vi "Periodic Tasks.vi"(8 "error in":errorcluster) -> ()   [LabVIEW 2017]
doc: "This VI runs in parallel to other tasks. It can contain as many user-defined periodic loops as you need. These can carry out PID or other sorts of timed response."
uses:
  <vilib>/Rock Robotics/WPI/Utilities/WPI_GetSetVariantRefNum.vi
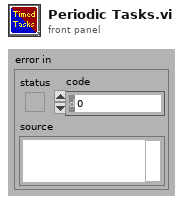
[diagram p1: front panel]
types:
  T1 = typedef "WPI_JoystickDevRef.ctl" = cluster{"Device":T2}
  T2 = typedef "WPI_JoystickDeviceEnum.ctl" = enum16{"USB 0", "USB 1", "USB 2", "USB 3", "USB 4", "USB 5"}
  T3 = typedef "WPI_RobotDriveDevRef.ctl" = cluster{"DevStatus":errorcluster, "Motors[]":T4[], "Square Inputs":bool, "Max Output":dbl}
  T4 = typedef "WPI_MotorControlDeviceRef.ctl" = cluster{"DeviceStatus":errorcluster, "Type":T5, "PWM":cluster{"PWM Channel":T6, "DeadBand":T7}, "CAN":cluster{"Device Number":u8, "SetOutput VI Ref":variant, "GetOutput VI Ref":variant, "Enable VI Ref":variant, "Disable VI Ref":variant, "Data":variant}, "Invert":bool, "DIO PWM":cluster{"PWM \"Enable\" Channel":T6, "DIOChannel":T8, "PWM Rate":dbl}}
  T5 = typedef "WPI_MotorControlType.ctl" = enum16{"PWM", "CAN", "DIO PWM"}
  T6 = typedef "FPGA_DIOPWMChannel.ctl" = enum8{"PWM 0", "PWM 1", "PWM 2", "PWM 3", "PWM 4", "PWM 5", "PWM 6", "PWM 7", "PWM 8", "PWM 9", "PWM MXP 0", "PWM MXP 1", "PWM MXP 2", "PWM MXP 3", "PWM MXP 4", "PWM MXP 5", "PWM MXP 6", "PWM MXP 7", "PWM MXP 8", "PWM MXP 9", "Invalid"}
  T7 = typedef "WPI_PWMDeadband.ctl" = cluster{"Name":string, "maxPositivePwm":i32, "minPositivePwm":i32, "centerPwm":i32, "maxNegativePwm":i32, "minNegativePwm":i32, "angularRange":u16}
  T8 = typedef "FPGA_DIOChannel.ctl" = enum8{"DIO 0", "DIO 1", "DIO 2", "DIO 3", "DIO 4", "DIO 5", "DIO 6", "DIO 7", "DIO 8", "DIO 9", "DIO MXP 0", "DIO MXP 1", "DIO MXP 2", "DIO MXP 3", "DIO MXP 4", "DIO MXP 5", "DIO MXP 6", "DIO MXP 7", "DIO MXP 8", "DIO MXP 9", "DIO MXP 10", "DIO MXP 11", "DIO MXP 12", "DIO MXP 13", "DIO MXP 14", "DIO MXP 15", "SPI Port CS1", "SPI Port CS2", "SPI Port CS3", "SPI Port MISO", "SPI Port MOSI", "Invalid"}
  T9 = cluster{"JoystickDevRef":T1, "RobotDriveDevRef":T3}
  T10 = typedef "WPI_I2CDevRef.ctl" = cluster{"DevStatus":errorcluster, "Device Address":u8, "Handle":i32, "I2C Bus":T11}
  T11 = typedef "i2c_bus.ctl" = enum16{"I2C On-Board", "I2C MXP", "Invalid"}
  T12 = typedef "WPI_DriverStationRobotMode2.ctl" = enum16{"Autonomous Disabled", "Autonomous Enabled", "Teleop Disabled", "Teleop Enabled", "Disconnected", "Finish", "Test Disabled", "Test Enabled", "Emergency Stopped"}
  T13 = typedef "WPI_DriverStationAllianceInfo.ctl" = enum16{"Red", "Blue", "Invalid"}
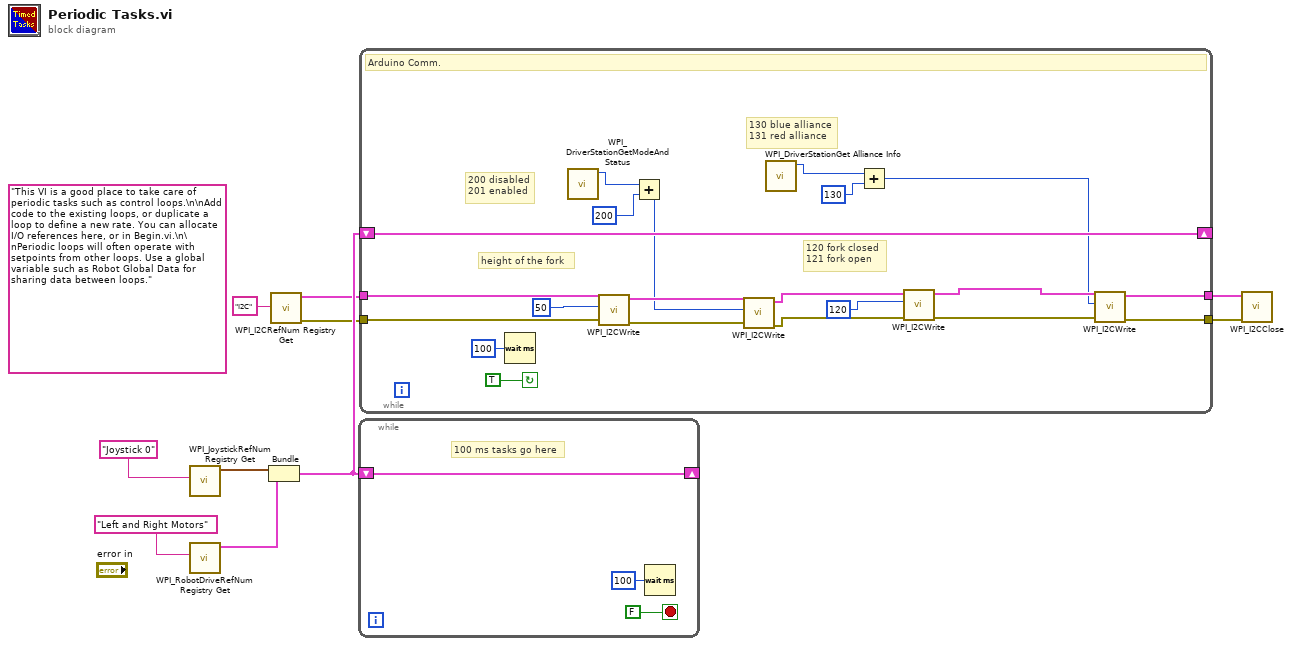
[diagram p0: block diagram]
diagram:
  (unwired) "This VI is a good place to take care of periodic tasks such as control loops.\n\nAdd code to the existing loops, or duplicate a loop to define a new rate. You can allocate I/O references here, or in Begin.vi.\n\nPeriodic loops will often operate with setpoints from other loops. Use a global variable such as Robot Global Data for sharing data between loops."
  n1 = call <vilib>:"WPI_JoystickRefNum Registry Get.vi"("refnum name"="Joystick 0") -> ("JoystickDevRef"=w8:T1)  [unwired: 1 in, 9 out]
  n2 = call <vilib>:"WPI_RobotDriveRefNum Registry Get.vi"("refnum name"="Left and Right Motors") -> ("RobotDriveDevRef"=w7:T3)  [unwired: 1 in, 9 out]
  n3 = Bundle("JoystickDevRef"=w8, "RobotDriveDevRef"=w7) -> (w6:T9)  [unwired: 1 out]
  n4 = call <vilib>:"WPI_I2CRefNum Registry Get.vi"("refnum name"="I2C") -> ("error out"=w4:errorcluster, "I2CDevRef"=w3:T10)  [unwired: 9 in]
  n5 = while {
    shift-right: [w11] -> _
    shift-left: w6 -> [w11]
    stop <- FALSE stop-if-true
    # "100 ms tasks go here"
    n6 = Wait (ms)(milliseconds to wait=u32 100) -> ()  [unwired: 1 out]
  }
  n7 = while {
    shift-right: [w32] -> _
    shift-left: w6 -> [w32]
    tunnel: w4 -> [w20]
    tunnel: w3 -> [w21]
    tunnel: [w31] -> w1
    tunnel: [w30] -> w2
    stop <- TRUE continue-if-true
    # "130 blue alliance\n131 red alliance"
    # "120 fork closed\n121 fork open"
    # "200 disabled\n201 enabled"
    # "height of the fork"
    # "Arduino Comm."
    n8 = Wait (ms)(milliseconds to wait=u32 100) -> ()  [unwired: 1 out]
    n9 = call <vilib>:"WPI_DriverStationGetModeAndStatus.vi"() -> ("Robot Mode"=w16:T12)  [unwired: 10 in, 1 out]
    n10 = call <vilib>:"WPI_I2CWrite.vi"("error in (no error)"=w20, "I2CRegister"=u8 50 ("number"), "I2CDevRef"=w21) -> ("error out"=w26:errorcluster, "I2CDevRef"=w29:T10)  [unwired: 7 in]
    n11 = Add(x=w16, y=200) -> (x+y=w14:i32)
    n12 = call <vilib>:"WPI_I2CWrite.vi"("error in (no error)"=w26, "I2CRegister"=w14, "I2CDevRef"=w29) -> ("error out"=w25:errorcluster, "I2CDevRef"=w28:T10)  [unwired: 7 in]
    n13 = call <vilib>:"WPI_DriverStationGet Alliance Info.vi"() -> ("Alliance"=w19:T13)  [unwired: 6 in, 5 out]
    n14 = Add(x=w19, y=130) -> (x+y=w17:i32)
    n15 = call <vilib>:"WPI_I2CWrite.vi"("error in (no error)"=w25, "I2CRegister"=u8 120 ("number"), "I2CDevRef"=w28) -> ("error out"=w24:errorcluster, "I2CDevRef"=w27:T10)  [unwired: 7 in]
    n16 = call <vilib>:"WPI_I2CWrite.vi"("error in (no error)"=w24, "I2CRegister"=w17, "I2CDevRef"=w27) -> ("error out"=w31:errorcluster, "I2CDevRef"=w30:T10)  [unwired: 7 in]
  }
  n17 = call <vilib>:"WPI_I2CClose.vi"("error in (no error)"=w1, "I2CDevRef"=w2) -> ()  [unwired: 9 in, 1 out]
